vi "SWITCH Action-Status Range.vi"(8 "error in (no error)":errorcluster, 10 "Message Data":variant, 11 "Data Cluster in":T1={"Tango HW"={"VISA resource"="", "Baud Rate (115200)"=2, "lAnInterfaceType"=0, "bAShowProt"=15}, "Writer Queue"=refnum, "Status"=FALSE, "Abs Position"=[], "Axis Velocity"={"dX"=0.0, "dY"=0.0, "dZ"=0.0, "dA"=0.0}, "acceleration "=0.0, "Z direction"=enum."Up", "Position Mode"="", "plLSID"=0}) -> (0 "error out":errorcluster, 3 "Data Cluster out":T1={"Tango HW"={"VISA resource"="", "Baud Rate (115200)"=2, "lAnInterfaceType"=0, "bAShowProt"=15}, "Writer Queue"=refnum, "Status"=FALSE, "Abs Position"=[], "Axis Velocity"={"dX"=0.0, "dY"=0.0, "dZ"=0.0, "dA"=0.0}, "acceleration "=0.0, "Z direction"=enum."Up", "Position Mode"="", "plLSID"=0})   [LabVIEW 2020, in "MOTOR.lvlib"]
uses:
  MOTOR.lvlib
  PS Hardware Configuration.ctl
  support/Message Queue/Message Cluster.ctl
  support/HW Message Cluster.ctl
  support/PCT FGV CMD.ctl
  support/Message Queue/Enqueue Message (Single).vi
  support/Message Queue/Message Queue.lvlib
  <instrlib>/Tango_DLL/Tango_DLL.lvlib
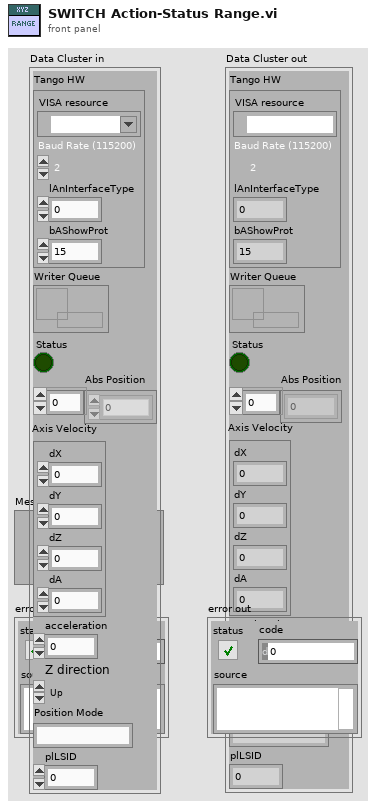
[diagram p1: front panel]
types:
  T1 = typedef "MOTOR.lvlib/PS Hardware Configuration.ctl" = cluster{"Tango HW":cluster{"VISA resource":refnum<visa-resource-name>, "Baud Rate (115200)":i32, "lAnInterfaceType":i32, "bAShowProt":i32}, "Writer Queue":refnum<queue>, "Status":bool, "Abs Position":i32[], "Axis Velocity":cluster{"dX":dbl, "dY":dbl, "dZ":dbl, "dA":dbl}, "acceleration ":dbl, "Z direction":enum16{"Up", "Down"}, "Position Mode":string, "plLSID":i32}
  T2 = typedef "PCT FGV CMD.ctl" = enum16{"INIT", "GET", "SET"}
  T3 = typedef "Message Queue.lvlib/HW Message Cluster.ctl" = cluster{"Writer Queue":refnum<queue>, "Writer Data":T4}
  T4 = typedef "Message Queue.lvlib/Message Cluster.ctl" = cluster{"Message":string, "Message Data":variant}
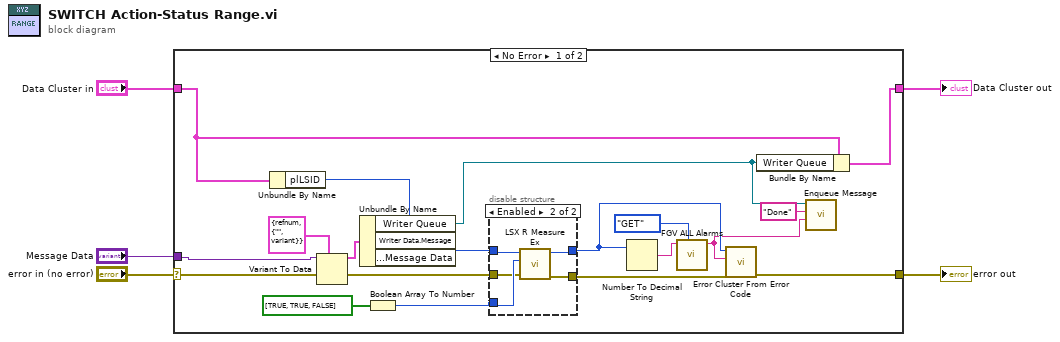
[diagram p0: block diagram]
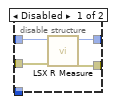
[diagram p2: hidden frame]
diagram:
  n1 = case shown="No Error" "error in (no error)" {
    selector: "error in (no error)" -> [w13 w32]
    tunnel: "Message Data" -> [w18 _]
    tunnel: [w19 w33] -> w4
    tunnel: "Data Cluster in" -> [w20 w33]
    tunnel: [w12 w32] -> w2
    frame No Error {
      n2 = Unbundle By Name(w20) -> ("plLSID"=w17:i32)
      n3 = Variant To Data(type=T3 {"Writer Queue"=refnum, "Writer Data"={"Message"="", "Message Data"=variant}}, Variant=w18) -> (data=w21:T3)  [unwired: 1 in, 1 out]
      n4 = Unbundle By Name(w21) -> ("Writer Queue"=w11:refnum<queue>)  [unwired: 2 out]
      n5 = Boolean Array To Number(Boolean array=bool[] [TRUE, TRUE, FALSE]) -> (number=w6:u32)
      n6 = disable-structure shown="Enabled" {
        disable-tunnel: w17 -> [w26 w31]
        disable-tunnel: [w25 w27] -> w14
        disable-tunnel: w13 -> [w24 w28]
        disable-tunnel: [w23 w30] -> w9
        disable-tunnel: w6 -> [_ w29]
        frame Disabled {
          n7 = call <instrlib>:"LSX R Measure.vi"("error in (no error)"=w24, "lLSID"=w26) -> ("error out"=w25:errorcluster, "function return"=w23:i32)  [unwired: 8 in]
        }
        frame Enabled {
          n8 = call <instrlib>:"LSX R Measure Ex.vi"("error in (no error)"=w28, "lFlags"=w29, "lLSID"=w31) -> ("error out"=w27:errorcluster, "function return"=w30:i32)  [unwired: 7 in]
        }
      }
      n9 = Number To Decimal String(number=w9) -> (decimal integer string=w15:string)  [unwired: 1 in]
      n10 = call "FGV ALL Alarms.vi"("CMD"=PCT_FGV_CMD."GET", "name"=w15) -> ("Alarm MSG out"=w8:string)  [unwired: 8 in, 1 out]
      n11 = call <vilib>:"Error Cluster From Error Code.vi"("error in (no error)"=w14, "error message (\"\")"=w8, "error code (0)"=w9) -> ("error out"=w12:errorcluster)  [unwired: 6 in]
      n12 = Bundle By Name(cluster=w20, "Writer Queue"=w11) -> (w19:T1)
      n13 = call-poly "Enqueue Message.vi"("Message Data"=w8, "Message"="Done", "Message Queue"=w11) -> ()  [unwired: 7 in, 2 out]
    }
    frame Error {
    }
  }
  "Data Cluster out" <- w4
  "error out" <- w2
